vi "Decrement Date.vi"(8 "error in (no error)":errorcluster, 11 "Budgetizer in":refnum<class "Budgetizer.lvclass">) -> (0 "error out":errorcluster, 3 "Budgetizer out":refnum<class "Budgetizer.lvclass">)   [LabVIEW 2018, in "Budgetizer.lvclass"]
uses:
  Budgetizer.lvclass
  Budgetizer.lvclass/Budgetizer.ctl
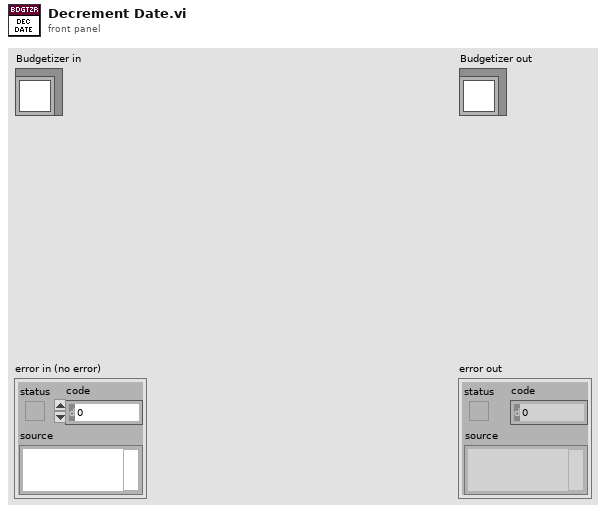
[diagram p1: front panel]
types:
  T1 = enum16{"January", "February", "March", "April", "May", "June", "July", "August", "September", "October", "November", "December"}
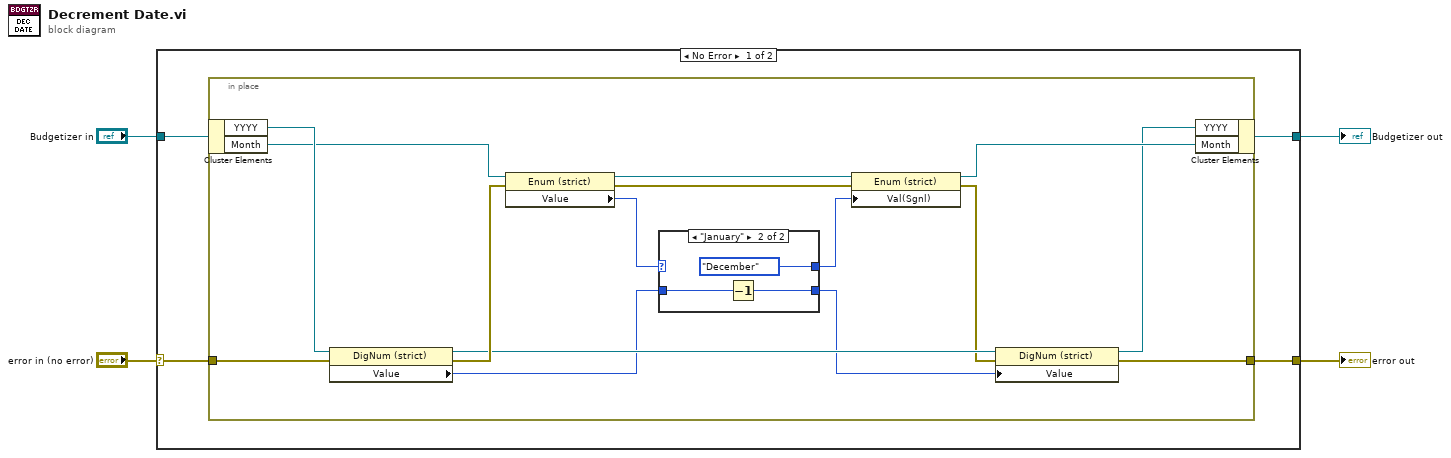
[diagram p0: block diagram]
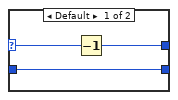
[diagram p2: hidden frame]
diagram:
  n1 = case shown="No Error" "error in (no error)" {
    selector: "error in (no error)" -> [w7 w31]
    tunnel: [w5 w31] -> w1
    tunnel: [w6 w30] -> w2
    tunnel: "Budgetizer in" -> [w8 w30]
    frame No Error {
      n2 = in-place {
        in-place-border: w7 -> [w21]
        in-place-border: [w13] -> w5
        n3 = in-place-cluster #1(w8) -> ("YYYY"=w22:refnum<vi>, "Month"=w20:refnum<vi>)
        n4 = property on="Property Node" class="DigNum (strict)"(reference=w22, error in=w21) -> (reference out=w16:refnum<vi>, error out=w23:errorcluster, "Value"=w11:i32)
        n5 = property on="Property Node" class="Enum (strict)"(reference=w20, error in=w23) -> (reference out=w18:refnum<vi>, error out=w19:errorcluster, "Value"=w12:T1)
        n6 = case shown="\"January\"" w12 {
          selector: w12 -> [w26 _]
          tunnel: w11 -> [w25 w28]
          tunnel: [w25 w27] -> w9
          tunnel: [w24 T1."December"] -> w10
          frame Default {
            n7 = Decrement(x=w26) -> (x-1=w24:T1)
          }
          frame "January" {
            n8 = Decrement(x=w28) -> (x-1=w27:i32)
          }
        }
        n9 = property on="Property Node" class="Enum (strict)"(reference=w18, error in=w19, "Val(Sgnl)"=w10) -> (reference out=w17:refnum<vi>, error out=w15:errorcluster)
        n10 = property on="Property Node" class="DigNum (strict)"(reference=w16, error in=w15, "Value"=w9) -> (reference out=w14:refnum<vi>, error out=w13:errorcluster)
        n11 = in-place-cluster #1("YYYY"=w14, "Month"=w17) -> (w6:refnum<class "Budgetizer.lvclass">)
      }
    }
    frame Error {
    }
  }
  "error out" <- w1
  "Budgetizer out" <- w2
